vi "AddTestMethod_Item_CanDragToProjectWindow.vi"(10 "DropTarget":T1, 11 "Object":T1) -> (3 "CanDrag":bool)   [LabVIEW 2013]
uses:
  <resource>/Framework/Providers/API/ItemRef.ctl
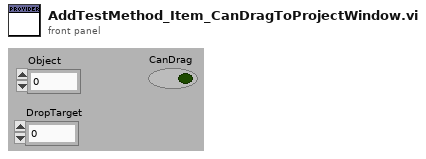
[diagram p1: front panel]
types:
  T1 = typedef "ItemRef.ctl" = u64
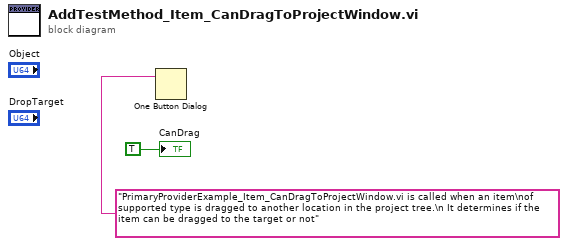
[diagram p0: block diagram]
diagram:
  n1 = One Button Dialog(message="PrimaryProviderExample_Item_CanDragToProjectWindow.vi is called when an item\nof supported type is dragged to another location in the project tree.\n It determines if the item can be dragged to the target or not") -> ()  [unwired: 1 in, 1 out]
  "CanDrag" <- TRUE ("CanDrag")
